vi "UART_Help.vi"(8 "error in (no error)":errorcluster caption="错误输入（无错误）", 9 "baud rate (115200)":u32=115200 caption="波特率(115200)", 10 "地址":u8=1, 11 "BASE_COM":refnum<visa-resource-name>="COM4") -> (0 "error out":errorcluster caption="错误输出", 1 "retStr":string, 2 "OK":bool, 3 "BASE_COM_OUT":refnum<visa-resource-name>)   [LabVIEW 2015, in "UARTCOM.lvlib"]
uses:
  UARTCOM.lvlib
  <vilib>/Instr/_visa.llb/VISA Configure Serial Port (Instr).vi
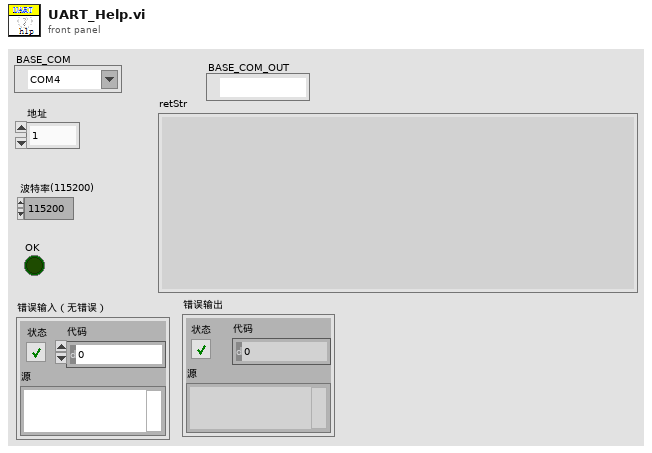
[diagram p1: front panel]
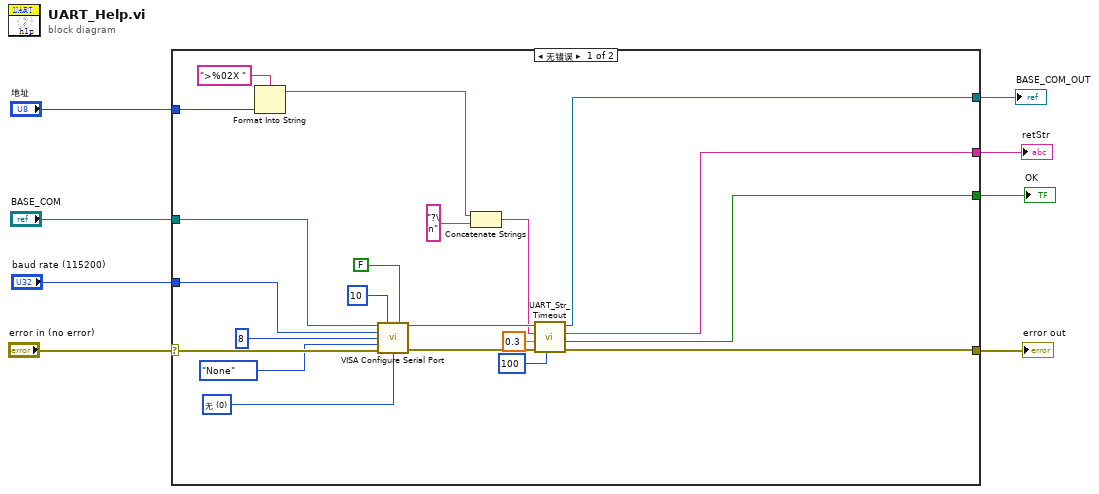
[diagram p0: block diagram]
diagram:
  n1 = case shown="无错误" "error in (no error)" {
    selector: "error in (no error)" -> [w29 w31]
    tunnel: [w14 w31] -> w7
    tunnel: "BASE_COM" -> [w20 w30]
    tunnel: "baud rate (115200)" -> [w26 _]
    tunnel: [w12 _] -> w4
    tunnel: "地址" -> [w19 _]
    tunnel: [w11 _] -> w2
    tunnel: [w9 w30] -> w1
    frame No Error {
      w23 = u16 0 items=["无", "XON/XOFF", "RTS/CTS", "XON/XOFF & RTS/CTS", "DTR/DSR", "XON/XOFF & DTR/DSR"] ("flow control (0:none)")
      n2 = Format Into String(format string=">%02X ", w19) -> (resulting string=w15:string)  [unwired: 2 in, 1 out]
      n3 = call-poly "VISA Configure Serial Port"("VISA resource name"=w20, "timeout (10sec)"=u32 10, "Enable Termination\nChar (T)"=FALSE ("Enable Termination\nChar (T)"), "baud rate (9600)"=w26, "data bits (8)"=u16 8, "parity (0:none)"=enum16{"None", "Odd", "Even", "Mark", "Space"}."None", "error in (no error)"=w29, "flow control (0:none)"=w23) -> ("VISA resource name out"=w21:refnum<visa-resource-name>, "error out"=w22:errorcluster)  [unwired: 6 in]
      n4 = Concatenate Strings(w15, "?\n" ("写入字符串")) -> (w16:string)
      n5 = call "UART_Str_Timeout.vi"("行数量"=u32 100, "error in (no error)"=w22, "超时s"=0.3, "写入字符串"=w16, "BASE_COM"=w21) -> ("error out"=w14:errorcluster, "OK"=w12:bool, "读取字符串"=w11:string, "BASE_COM_OUT"=w9:refnum<visa-resource-name>)  [unwired: 2 in, 1 out]
    }
    frame Error {
    }
  }
  "error out" <- w7
  "OK" <- w4
  "retStr" <- w2
  "BASE_COM_OUT" <- w1
